vi "while_v0_v6.vi"() -> ()   [LabVIEW 2009]
panel:
  in  "Delay intre doua puncte(ms)":dbl(slide)=21.20253164556962 scale=0.0..100.0
  in  "Grade intre 2 puncte":dbl(knob)=8.811117808929394 scale=0.1..10.0
  out "Waveform Chart":dbl(graph)=0.9875126612016873
  in  "stop":bool
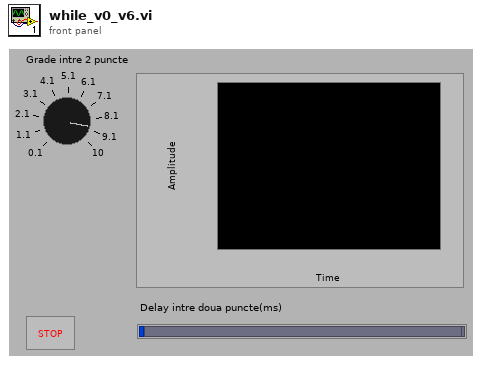
[diagram p1: front panel]
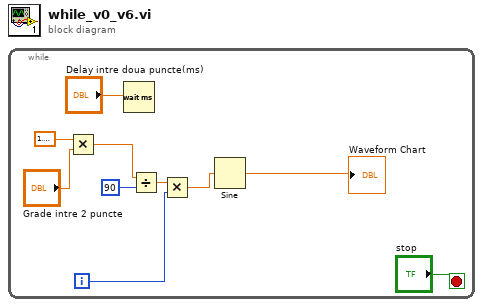
[diagram p0: block diagram]
diagram:
  n1 = while {
    i -> [w3]
    stop <- "stop" stop-if-true
    n2 = Multiply(x=1.5707963267948966, y="Grade intre 2 puncte") -> (x*y=w5:dbl)
    n3 = Wait (ms)(milliseconds to wait="Delay intre doua puncte(ms)") -> ()  [unwired: 1 out]
    n4 = Divide(x=w5, y=90) -> (x/y=w4:dbl)
    n5 = Multiply(x=w4, y=w3) -> (x*y=w2:dbl)
    n6 = Sine(x=w2) -> (sin(x)=→"Waveform Chart":dbl)
  }
